vi "Autobalance Results Display.vi"(3 "error in (no error)":errorcluster) -> (10 "error out":errorcluster)   [LabVIEW 2009]
uses:
  lib/Data Access Objects/Metadata/LBCB Number.ctl
  lib/Data Access Objects/Metadata/DAO Actions.ctl
  lib/Global Data/Actuator Measurment Actions.ctl
panel:
  out "Prev Cmd L1":dbl[](array[numeric]) caption="Previous Command Differences"
  out "Prev Cmd  L2":dbl[](array[numeric]) caption="Previous Command Differences"
  out "Actuator DOF Labels 2":string[](array[string])=["X1", "X2", "Y1", "Z1", "Z2", "Z3"]
  out "AB Diff L2":dbl[](array[numeric]) caption="Autobalance Differences"
  out "PC Diff L2":dbl[](array[numeric]) caption="Previous Command Differences"
  out "Actuator DOF Labels":string[](array[string])=["X1", "X2", "Y1", "Z1", "Z2", "Z3"]
  in  "Ok":bool
  out "AB Diff L1":dbl[](array[numeric]) caption="Autobalance Differences"
  out "PC Diff L1":dbl[](array[numeric]) caption="Previous Command Differences"
  # "LBCB 1"
  # "LBCB 2"
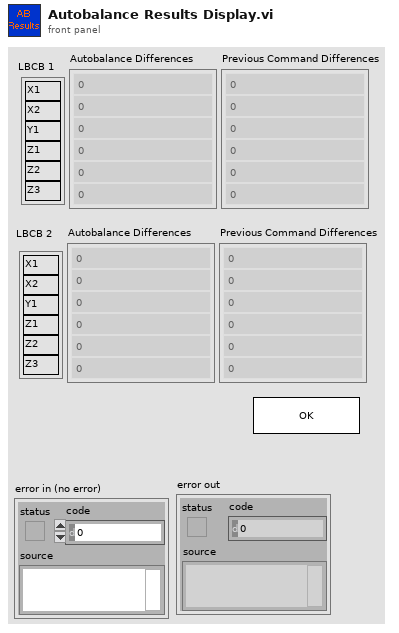
[diagram p1: front panel]
types:
  T1 = typedef "LBCB Number.ctl" = enum16{"LBCB1", "LBCB2"}
  T2 = typedef "DAO Actions.ctl" = enum16{"Init", "Get", "Set"}
  T3 = typedef "Actuator Point.ctl" = cluster{"X1":dbl, "X2":dbl, "Y1":dbl, "Z1":dbl, "Z2":dbl, "Z3":dbl}
  T4 = typedef "Actuator Measurment Actions.ctl" = enum16{"Set  Data", "Get", "Init"}
  T5 = typedef "Actuator DataType.ctl" = cluster{"LVDTs":dbl[], " Commands":dbl[], "Load Cells":dbl[], "Servo":dbl[]}
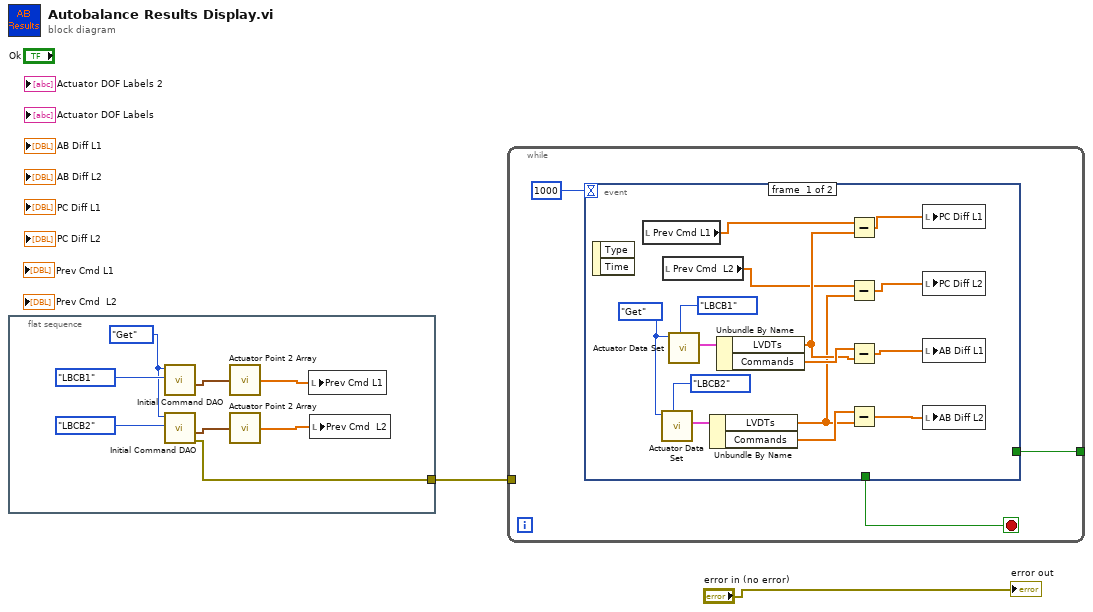
[diagram p0: block diagram]
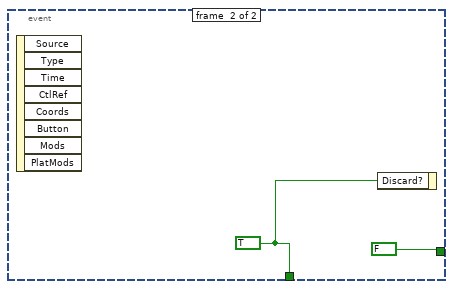
[diagram p2: hidden frame]
diagram:
  n1 = flat-sequence {
    tunnel: [w3] -> w1
    frame #0 {
      w5 = DAO_Actions."Get" ("DAO Actions")
      n2 = call "Initial Command DAO.vi"("LBCB Number"=LBCB_Number."LBCB1" ("Selected LBCB"), "DAO Actions"=w5) -> ("Command Out"=w9:T3)  [unwired: 2 in, 7 out]
      n3 = call "Initial Command DAO.vi"("LBCB Number"=LBCB_Number."LBCB2" ("Selected LBCB"), "DAO Actions"=w5) -> ("error out"=w3:errorcluster, "Command Out"=w6:T3)  [unwired: 2 in, 6 out]
      n4 = call "Actuator Point 2 Array.vi"("Actuator Point"=w9) -> ("Array"=w8:dbl[])
      n5 = call "Actuator Point 2 Array.vi"("Actuator Point"=w6) -> ("Array"=w4:dbl[])
      n6 = local write "Prev Cmd L1"(w8) -> ()
      n7 = local write "Prev Cmd  L2"(w4) -> ()
    }
  }
  n8 = while {
    tunnel: [w11] -> _
    tunnel: w1 -> [_]
    stop <- w12 stop-if-true
    n9 = event shown="[1] \"Ok\": Mouse Down?" {
      selector: _ -> [_ _]
      dyn-events: _ -> [_ _]
      timeout: 1000 -> [_ _]
      tunnel: [_ w29] -> w12
      tunnel: [_ FALSE] -> w11
      event #0 {
        w22 = Actuator_Measurment_Actions."Get" ("Measurement Actions")
        n10 = event-data() -> ()  [unwired: 3 out]
        n11 = local read "Prev Cmd L1"() -> (w18:dbl[])
        n12 = call "Actuator Data Set.vi"("Selected LBCB"=LBCB_Number."LBCB2", "Measurement Actions"=w22) -> ("Actuator Data Out"=w24:T5)  [unwired: 3 in, 6 out]
        n13 = local read "Prev Cmd  L2"() -> (w16:dbl[])
        n14 = call "Actuator Data Set.vi"("Selected LBCB"=LBCB_Number."LBCB1", "Measurement Actions"=w22) -> ("Actuator Data Out"=w28:T5)  [unwired: 3 in, 6 out]
        n15 = Unbundle By Name(w24) -> ("LVDTs"=w15:dbl[], "Commands"=w21:dbl[])
        n16 = Unbundle By Name(w28) -> ("LVDTs"=w17:dbl[], "Commands"=w27:dbl[])
        n17 = Subtract(x=w18, y=w17) -> (x-y=w19:dbl[])
        n18 = Subtract(x=w16, y=w15) -> (x-y=w14:dbl[])
        n19 = Subtract(x=w27, y=w17) -> (x-y=w26:dbl[])
        n20 = Subtract(x=w21, y=w15) -> (x-y=w20:dbl[])
        n21 = local write "PC Diff L1"(w19) -> ()
        n22 = local write "PC Diff L2"(w14) -> ()
        n23 = local write "AB Diff L1"(w26) -> ()
        n24 = local write "AB Diff L2"(w20) -> ()
      }
      event #1 {
        w29 = TRUE
        n25 = event-data() -> ()  [unwired: 9 out]
        n26 = event-data("Discard?"=w29) -> ()  [unwired: 1 in, 1 out]
      }
    }
  }
  "error out" <- "error in (no error)"
